vi "rotate sorting options.vi"(8 "error in":errorcluster, 10 "Column":i32, 11 "taglist":refnum<data-value>) -> (0 "error out":errorcluster)   [LabVIEW 2013, in "PL Framework Configuration Tool.lvlib" / "EngineTags.lvclass"]
uses:
  EngineTags.lvclass
  EngineTags.lvclass/EngineTags.ctl
  sorting type.ctl
  Read Sorting Enabled.vi
  Read Sorting Column.vi
  Write Sorting Enabled.vi
  Write Sorting Column.vi
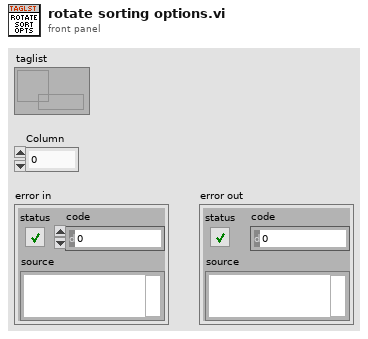
[diagram p1: front panel]
types:
  T1 = typedef "PL Framework Configuration Tool.lvlib/EngineTags.lvclass/sorting type.ctl" = enum16{"none", "asc", "desc"}
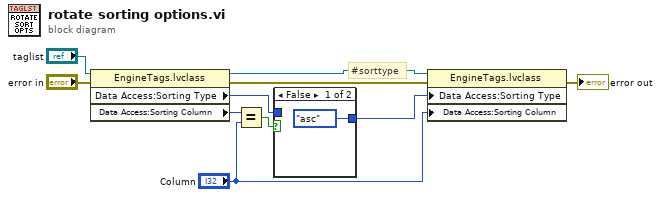
[diagram p0: block diagram]
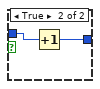
[diagram p2: hidden frame]
diagram:
  # "#sorttype"
  n1 = property class="EngineTags.lvclass"(reference="taglist", error in="error in") -> (reference out=w3:refnum<data-value>, error out=w4:errorcluster, "Data Access:Sorting Type"=w9:T1, "Data Access:Sorting Column"=w7:i32)
  n2 = Equal?(x=w7, y="Column") -> (x = y?=w8:bool)
  n3 = case shown="False" w8 {
    tunnel: w9 -> [_ w13]
    tunnel: [sorting_type."asc" ("Sorting Type") w12] -> w10
    frame False {
    }
    frame True {
      n4 = Increment(x=w13) -> (x+1=w12:T1)
    }
  }
  n5 = property class="EngineTags.lvclass"(reference=w3, error in=w4, "Data Access:Sorting Type"=w10, "Data Access:Sorting Column"="Column") -> (error out=→"error out":errorcluster)  [unwired: 1 out]
